vi "Linearization.vi"(1 "Input":dbl) -> (0 "Output":dbl)   [LabVIEW 2015]
uses:
  <vilib>/Analysis/polynomials.llb/Scalar Polynomial Evaluation (DBL).vi
  <vilib>/Analysis/NI_AALPro.lvlib
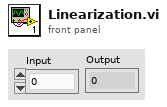
[diagram p1: front panel]
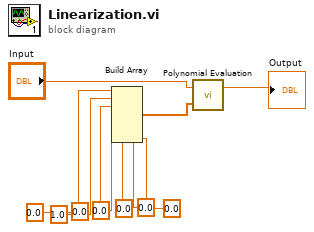
[diagram p0: block diagram]
diagram:
  n1 = Build Array(0.0 ("element"), 1.0 ("element"), 0.0 ("element"), 0.0 ("element"), 0.0 ("element"), 0.0 ("element"), 0.0 ("element")) -> (w10:dbl[])
  n2 = call-poly <vilib>:"Polynomial Evaluation.vi"("P(x)"=w10, "a"="Input") -> ("P(a)"=→"Output":dbl)  [unwired: 1 out]
